vi "SetPrecision.vi"(8 "error in":errorcluster, 10 "Precision":u8, 11 "RealMeasureLimit in":refnum<class "RealMeasureLimit.lvclass">) -> (0 "error out":errorcluster, 3 "RealMeasureLimit out":refnum<class "RealMeasureLimit.lvclass">)   [LabVIEW 2021, in "ProligentXMLGenerator.lvlib" / "RealMeasureLimit.lvclass"]
doc: "Real Measure Limit Lower Bound"
uses:
  RealMeasureLimit.lvclass
  RealMeasureLimit.lvclass/RealMeasureLimit.ctl
  RangeMeasureLimit/RangeMeasureLimit.lvclass
  Base/Decimal/Decimal.lvclass
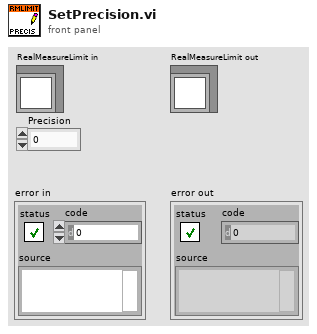
[diagram p1: front panel]
types:
  T1 = typedef "ProligentXMLGenerator.lvlib/RealMeasureLimit.lvclass/Data.ctl" = cluster{"LowerBound":refnum<class "Decimal.lvclass">, "HigherBound":refnum<class "Decimal.lvclass">}
  T2 = typedef "ProligentXMLGenerator.lvlib/RangeMeasureLimit.lvclass/ComparisonType.ctl" = enum16{"LowerBound <= X <= HigherBound", "LowerBound < X <= HigherBound", "LowerBound <= X < HigherBound", "LowerBound < X < HigherBound", "LowerBound <= X", "LowerBound < X", "X <= HigherBound", "X < HigherBound", "X == HigherBound", "X != HigherBound", "X <= LowerBound OR HigherBound <= X", "X < LowerBound OR HigherBound <= X", "X <= LowerBound OR HigherBound < X", "X < LowerBound OR HigherBound < X"}
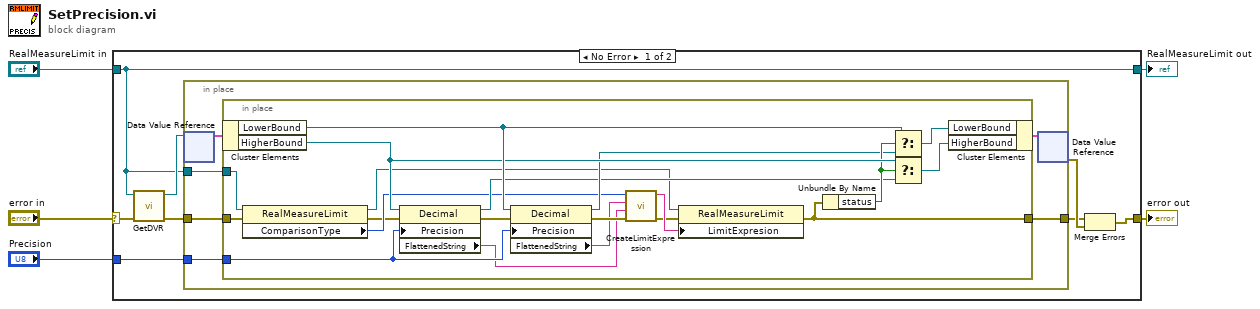
[diagram p0: block diagram]
diagram:
  n1 = case shown="No Error" "error in" {
    selector: "error in" -> [w7 w40]
    tunnel: "RealMeasureLimit in" -> [w6 w41]
    tunnel: [w12 w40] -> w3
    tunnel: "Precision" -> [w11 _]
    tunnel: [w6 w41] -> w1
    frame No Error {
      n2 = call "GetDVR.vi"("error in"=w7, "RealMeasureLimit"=w6) -> ("error out"=w10:errorcluster, "DVRReference"=w13:refnum<data-value>)  [unwired: 8 in]
      n3 = in-place "In Place Element Structure" {
        in-place-border: w11 -> [w19]
        in-place-border: w10 -> [w16]
        in-place-border: [w15] -> w8
        in-place-border: w6 -> [w14]
        n4 = in-place-dvr #1(w13) -> (w18:T1)  [unwired: 1 out]
        n5 = in-place "In Place Element Structure" {
          in-place-border: w19 -> [w34]
          in-place-border: w16 -> [w23]
          in-place-border: [w37] -> w15
          in-place-border: w14 -> [w24]
          n6 = in-place-cluster #2(w18) -> ("LowerBound"=w31:refnum<class "Decimal.lvclass">, "HigherBound"=w28:refnum<class "Decimal.lvclass">)
          n7 = property class="RealMeasureLimit"(reference=w24, error in=w23) -> (reference out=w21:refnum<class "RealMeasureLimit.lvclass">, error out=w20:errorcluster, "ComparisonType"=w22:T2)
          n8 = property class="Decimal"(reference=w28, error in=w20, "Precision"=w34) -> (reference out=w25:refnum<class "Decimal.lvclass">, error out=w36:errorcluster, "FlattenedString"=w33:string)
          n9 = property class="Decimal"(reference=w31, error in=w36, "Precision"=w34) -> (reference out=w26:refnum<class "Decimal.lvclass">, error out=w35:errorcluster, "FlattenedString"=w32:string)
          n10 = call "CreateLimitExpression.vi"("error in"=w35, "HigherBound"=w33, "LowerBound"=w32, "ComparisonType"=w22) -> ("error out"=w38:errorcluster, "LimitExpression"=w39:string)  [unwired: 6 in]
          n11 = property class="RealMeasureLimit"(reference=w21, error in=w38, "LimitExpresion"=w39) -> (error out=w37:errorcluster)  [unwired: 1 out]
          n12 = Unbundle By Name(w37) -> ("status"=w27:bool)
          n13 = Select(t=w31, s=w27, f=w26) -> (s? t:f=w30:refnum<class "Decimal.lvclass">)
          n14 = Select(t=w28, s=w27, f=w25) -> (s? t:f=w29:refnum<class "Decimal.lvclass">)
          n15 = in-place-cluster #2("LowerBound"=w30, "HigherBound"=w29) -> (w17:T1)
        }
        n16 = in-place-dvr #1(w17) -> (w9:errorcluster)  [unwired: 1 out]
      }
      n17 = Merge Errors(w8, w9) -> (w12:errorcluster)
    }
    frame Error {
    }
  }
  "error out" <- w3
  "RealMeasureLimit out" <- w1
